vi "FTW-Color-Hue to Color Component.vi"(1 "Hue Vars":cluster{"Var 1":dbl, "Var 2":dbl, "Hue":dbl}) -> (0 "Color Component Value":dbl)   [LabVIEW 2013]
doc: "Converts the Hue of an HSL (Hue, Saturation, Lumanence) color space color value into an 32 bit RGB (Red, Green, Blue) Color space 8 bit component value."
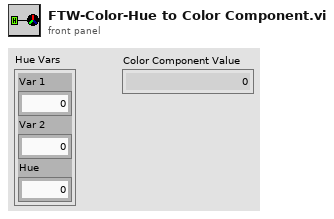
[diagram p1: front panel]
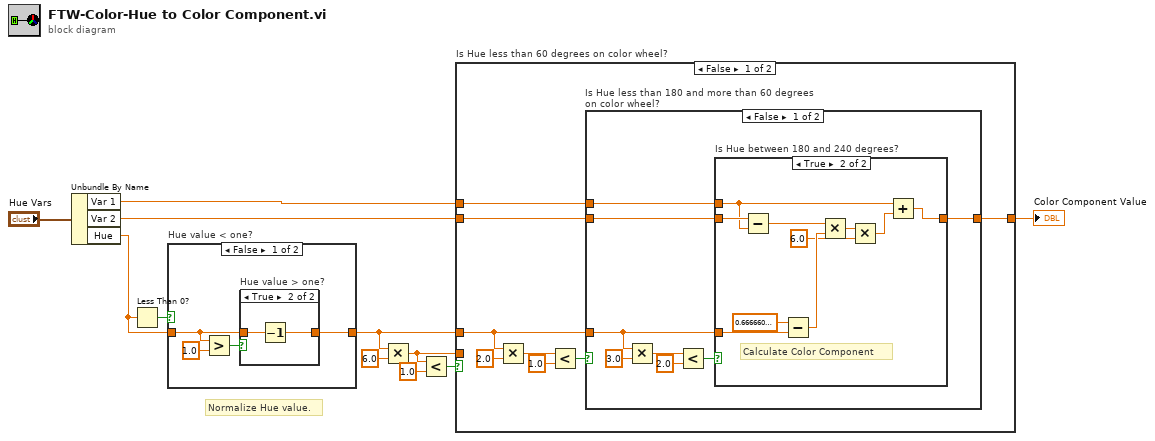
[diagram p0: block diagram]
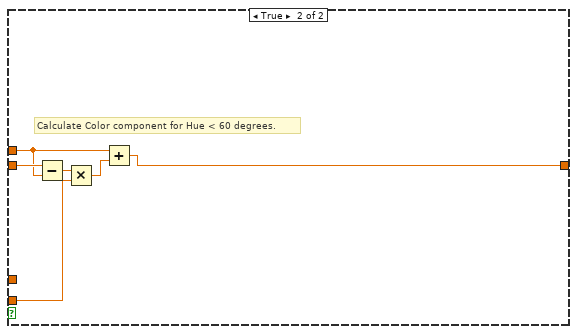
[diagram p4: hidden frame]
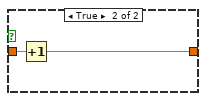
[diagram p6: hidden frame]
diagram:
  # "Normalize Hue value."
  n1 = Unbundle By Name("Hue Vars") -> ("Var 1"=w7:dbl, "Var 2"=w6:dbl, "Hue"=w5:dbl)
  n2 = Less Than 0?(x=w5) -> (x < 0?=w10:bool)
  n3 = case "Hue value < one?" shown="False" w10 {
    tunnel: w5 -> [w12 w20]
    tunnel: [w13 w19] -> w4
    frame False {
      n4 = Greater?(x=w12, y=1.0) -> (0:w14:bool)
      n5 = case "Hue value > one?" shown="True" w14 {
        tunnel: w12 -> [w16 w18]
        tunnel: [w16 w17] -> w13
        frame False {
        }
        frame True {
          n6 = Decrement(x=w18) -> (x-1=w17:dbl)
        }
      }
    }
    frame True {
      n7 = Increment(x=w20) -> (x+1=w19:dbl)
    }
  }
  n8 = Multiply(x=w4, y=6.0) -> (x*y=w2:dbl)
  n9 = Less?(x=w2, y=1.0) -> (x < y?=w3:bool)
  n10 = case "Is Hue less than 60 degrees on color wheel?" shown="False" w3 {
    tunnel: w7 -> [w23 w51]
    tunnel: w6 -> [w24 w54]
    tunnel: w4 -> [w21 _]
    tunnel: w2 -> [_ w53]
    tunnel: [w22 w50] -> w1
    frame False {
      n11 = Multiply(x=w21, y=2.0) -> (x*y=w26:dbl)
      n12 = Less?(x=w26, y=1.0) -> (x < y?=w25:bool)
      n13 = case "Is Hue less than 180 and more than 60 degrees on color wheel?" shown="False" w25 {
        tunnel: w21 -> [w29 _]
        tunnel: w24 -> [w32 w48]
        tunnel: w23 -> [w31 _]
        tunnel: [w30 w48] -> w22
        frame False {
          n14 = Multiply(x=w29, y=3.0) -> (x*y=w36:dbl)
          n15 = Less?(x=w36, y=2.0) -> (x < y?=w33:bool)
          n16 = case "Is Hue between 180 and 240 degrees?" shown="True" w33 {
            tunnel: w29 -> [_ w46]
            tunnel: w32 -> [_ w47]
            tunnel: w31 -> [w37 w41]
            tunnel: [w37 w38] -> w30
            frame False {
              # "Color Component is Var 1"
            }
            frame True {
              # "Calculate Color Component"
              n17 = Subtract(x=w47, y=w41) -> (x-y=w44:dbl)
              n18 = Subtract(x=0.6666600108146667, y=w46) -> (x-y=w43:dbl)
              n19 = Multiply(x=w44, y=w43) -> (x*y=w42:dbl)
              n20 = Multiply(x=w42, y=6.0 ("x")) -> (x*y=w39:dbl)
              n21 = Add(x=w41, y=w39) -> (x+y=w38:dbl)
            }
          }
        }
        frame True {
          # "Color Component is Var 2."
        }
      }
    }
    frame True {
      # "Calculate Color component for Hue < 60 degrees."
      n22 = Subtract(x=w54, y=w51) -> (x-y=w52:dbl)
      n23 = Multiply(x=w52, y=w53) -> (x*y=w49:dbl)
      n24 = Add(x=w51, y=w49) -> (x+y=w50:dbl)
    }
  }
  "Color Component Value" <- w1
